vi "IntakeForTime.vi"() -> ()   [LabVIEW 2017]
uses:
  Framework/Robot Global Data.vi
panel:
  in  "Time":u32
  in  "Speed":dbl
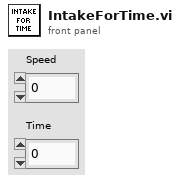
[diagram p1: front panel]
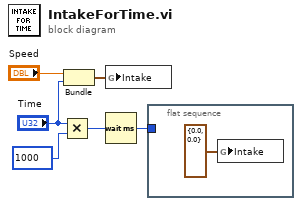
[diagram p0: block diagram]
diagram:
  n1 = Multiply(x="Time", y=u32 1000) -> (x*y=w5:u32)
  n2 = Bundle("Speed"="Speed", "Time"="Time") -> (w4:cluster{"Speed":dbl, "Time":u32})  [unwired: 1 in]
  n3 = global write "Robot Global Data.vi" "Intake"(w4) -> ()
  n4 = Wait (ms)(milliseconds to wait=w5) -> (millisecond timer value=w3:u32)
  n5 = flat-sequence {
    tunnel: w3 -> [_]
    frame #0 {
      n6 = global write "Robot Global Data.vi" "Intake"(cluster{"Drive Speed":dbl, "Drive Time":dbl} {"Drive Speed"=0.0, "Drive Time"=0.0} ("Drive")) -> ()
    }
  }
